vi "Close.vi"(7 "Server Alias":string, 8 "error in (no error)":errorcluster) -> (0 "error out":errorcluster)   [LabVIEW 2013, in "TS.lvlib"]
doc: "This VI stops the Server. Use this when you no longer need TestScript."
uses:
  TS.lvlib
  Private/Status Message.ctl
  LabVIEW Python Connector Message.ctl
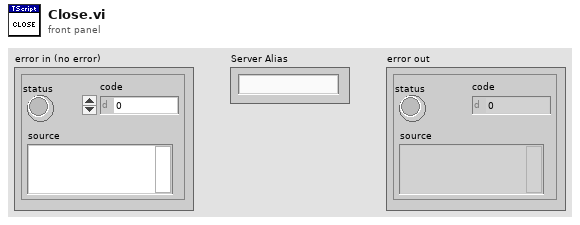
[diagram p1: front panel]
types:
  T1 = typedef "TS.lvlib/LabVIEW Python Connector Message.ctl" = cluster{"Command":string, "Data":string[], "Script ID":i64, "LabVIEW Server ID":string, "Python Message ID":i32}
  T2 = typedef "TS.lvlib/Status Message.ctl" = cluster{"Text":string, "Time":timestamp}
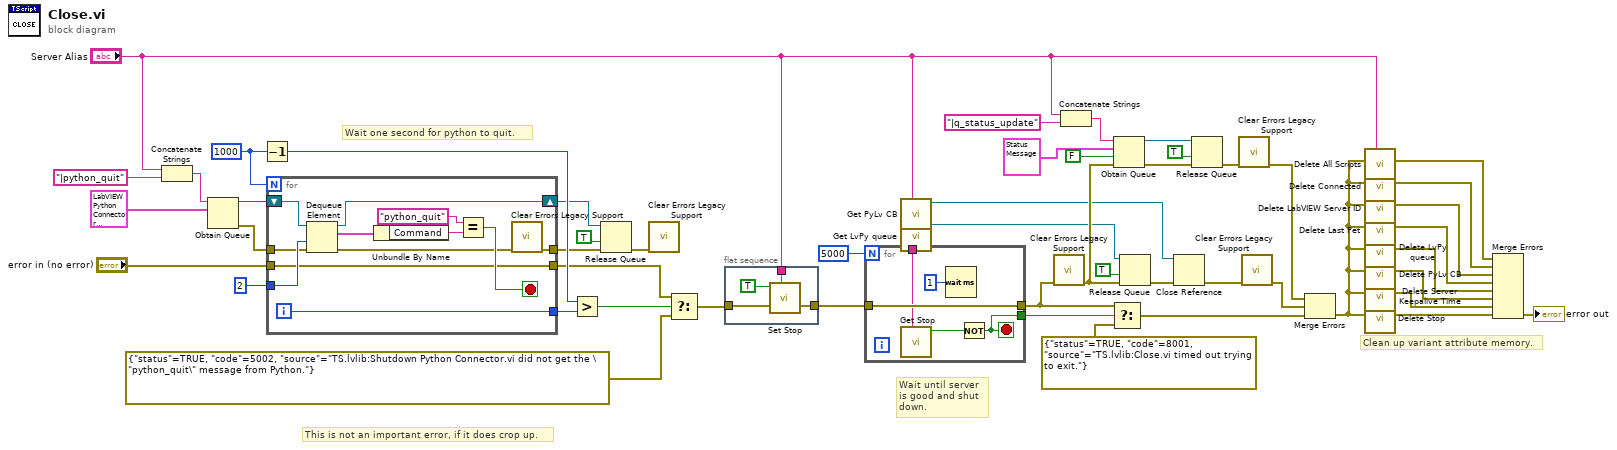
[diagram p0: block diagram]
diagram:
  w45 = 1000
  # "Clean up variant attribute memory."
  # "This is not an important error, if it does crop up."
  # "Wait one second for python to quit."
  # "Wait until server\nis good and shut\ndown."
  n1 = Concatenate Strings("Server Alias", "|python_quit" ("name (unnamed)")) -> (w3:string)
  n2 = Obtain Queue(name (unnamed)=w3, element data type=T1 {"Command"="zxcvbnm,", "Data"=["asdfghjk", "qwertyui"], "Script ID"=0, "LabVIEW Server ID"="zxcvbnm,", "Python Message ID"=0}) -> (queue out=w19:refnum<queue>, error out=w18:errorcluster)  [unwired: 3 in, 1 out]
  n3 = Decrement(x=w45) -> (x-1=w43:i32)
  n4 = for {
    N: w45 -> [_]
    tunnel: "error in (no error)" -> [w55]
    tunnel: 2 ("timeout in ms (-1)") -> [w62]
    tunnel: [w56] -> w44
    tunnel: [w55] -> w41
    shift-right: [w54] -> w36
    shift-left: w19 -> [w63]
    tunnel: [w53] -> w37
    tunnel: w18 -> [w52]
    i -> [w56]
    stop <- w58 stop-if-true
    n5 = Dequeue Element(queue=w63, timeout in ms (-1)=w62, error in (no error)=w52) -> (queue out=w54:refnum<queue>, element=w61:T1, error out=w57:errorcluster)  [unwired: 1 out]
    n6 = Unbundle By Name(w61) -> ("Command"=w60:string)
    n7 = Equal?(x="python_quit", y=w60) -> (x = y?=w58:bool)
    n8 = call "Clear Errors Legacy Support.vi"("error in (no error)"=w57) -> ("error out"=w53:errorcluster)  [unwired: 5 in, 1 out]
  }
  n9 = Greater?(x=w43, y=w44) -> (0:w42:bool)
  n10 = Release Queue(queue=w36, force destroy? (F)=TRUE, error in (no error)=w37) -> (error out=w35:errorcluster)  [unwired: 2 out]
  n11 = call "Clear Errors Legacy Support.vi"("error in (no error)"=w35) -> ()  [unwired: 5 in, 2 out]
  n12 = Select(t=w41, s=w42, f=errorcluster {"status"=TRUE, "code"=5002, "source"="TS.lvlib:Shutdown Python Connector.vi did not get the \"python_quit\" message from Python."}) -> (s? t:f=w39:errorcluster)
  n13 = flat-sequence {
    tunnel: w39 -> [w66]
    tunnel: [w66] -> w51
    tunnel: "Server Alias" -> [w64]
    frame #0 {
      n14 = call "Set Stop.vi"("Server Alias"=w64, "Stop"=TRUE) -> ()  [unwired: 9 in, 1 out]
    }
  }
  n15 = for {
    N: 5000 -> [_]
    tunnel: w51 -> [w71]
    tunnel: [w71] -> w33
    tunnel: [w69] -> w49
    tunnel: "Server Alias" -> [w67]
    stop <- w69 stop-if-true
    n16 = call "Get Stop.vi"("Server Alias"=w67) -> ("Stop"=w68:bool)  [unwired: 9 in, 1 out]
    n17 = Wait (ms)(milliseconds to wait=u32 1) -> ()  [unwired: 1 out]
    n18 = Not(x=w68) -> (.not. x?=w69:bool)
  }
  n19 = call "Get PyLv CB.vi"("Server Alias"="Server Alias") -> ("VI Refnum"=w17:refnum<vi>)  [unwired: 9 in, 1 out]
  n20 = call "Get LvPy queue.vi"("Server Alias"="Server Alias") -> ("LvPy queue"=w16:refnum<queue>)  [unwired: 9 in, 1 out]
  n21 = call "Clear Errors Legacy Support.vi"("error in (no error)"=w33) -> ("error out"=w22:errorcluster)  [unwired: 5 in, 1 out]
  n22 = Concatenate Strings("Server Alias", "|q_status_update" ("name (unnamed)")) -> (w2:string)
  n23 = Select(t=w33, s=w49, f=errorcluster {"status"=TRUE, "code"=8001, "source"="TS.lvlib:Close.vi timed out trying to exit."} ("error in (no error)")) -> (s? t:f=w48:errorcluster)
  n24 = Obtain Queue(name (unnamed)=w2, element data type=T2 {"Text"="", "Time"=timestamp(0 s since 1904-01-01)} ("Status Update Message"), create if not found? (T)=FALSE, error in (no error)=w22) -> (queue out=w24:refnum<queue>, error out=w25:errorcluster)  [unwired: 1 in, 1 out]
  n25 = Release Queue(queue=w16, force destroy? (F)=TRUE, error in (no error)=w22) -> (error out=w31:errorcluster)  [unwired: 2 out]
  n26 = Close Reference(reference=w17, error in (no error)=w31) -> (error out=w30:errorcluster)
  n27 = Release Queue(queue=w24, force destroy? (F)=TRUE, error in (no error)=w25) -> (error out=w23:errorcluster)  [unwired: 2 out]
  n28 = call "Clear Errors Legacy Support.vi"("error in (no error)"=w23) -> ("error out"=w14:errorcluster)  [unwired: 5 in, 1 out]
  n29 = call "Clear Errors Legacy Support.vi"("error in (no error)"=w30) -> ("error out"=w15:errorcluster)  [unwired: 5 in, 1 out]
  n30 = Merge Errors(w14, w15, w48) -> (w4:errorcluster)
  n31 = call "Delete All Scripts.vi"("Server Alias"="Server Alias", "Error In"=w4) -> ("Error Out"=w6:errorcluster)  [unwired: 9 in]
  n32 = call "Delete Connected.vi"("Server Alias"="Server Alias", "Error In"=w4) -> ("Error Out"=w7:errorcluster)  [unwired: 9 in]
  n33 = call "Delete LabVIEW Server ID.vi"("Server Alias"="Server Alias", "Error In"=w4) -> ("Error Out"=w8:errorcluster)  [unwired: 9 in]
  n34 = call "Delete Last Pet.vi"("Server Alias"="Server Alias", "Error In"=w4) -> ("Error Out"=w9:errorcluster)  [unwired: 9 in]
  n35 = call "Delete LvPy queue.vi"("Server Alias"="Server Alias", "Error In"=w4) -> ("Error Out"=w10:errorcluster)  [unwired: 9 in]
  n36 = call "Delete PyLv CB.vi"("Server Alias"="Server Alias", "Error In"=w4) -> ("Error Out"=w11:errorcluster)  [unwired: 9 in]
  n37 = call "Delete Server Keepalive Time.vi"("Server Alias"="Server Alias", "Error In"=w4) -> ("Error Out"=w12:errorcluster)  [unwired: 9 in]
  n38 = call "Delete Stop.vi"("Server Alias"="Server Alias", "Error In"=w4) -> ("Error Out"=w13:errorcluster)  [unwired: 9 in]
  n39 = Merge Errors(w6, w7, w8, w9, w10, w11, w12, w13) -> (→"error out":errorcluster)
